vi "SetSubMenuIconType.vi"(8 "error in (no error)":errorcluster, 10 "SubMenuIcon":T1, 11 "Menu in":refnum<class "Menu.lvclass">) -> (0 "error out":errorcluster, 3 "Menu out":refnum<class "Menu.lvclass">)   [LabVIEW 2021, in "Menu.lvlib" / "Menu.lvclass"]
uses:
  Menu.lvclass
  SubMenuIcon.ctl
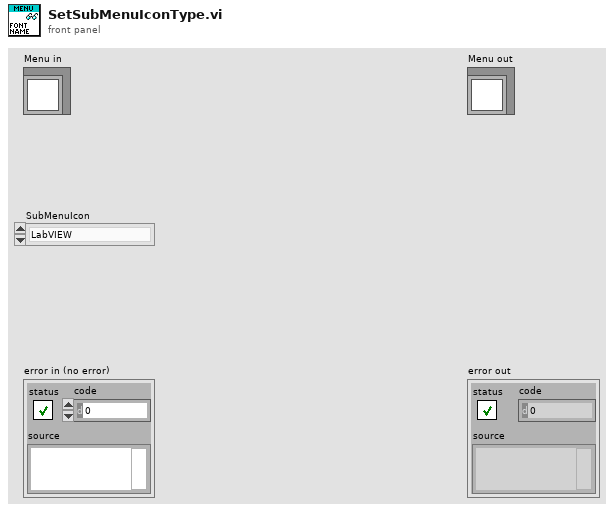
[diagram p1: front panel]
types:
  T1 = typedef "Menu.lvlib/Menu.lvclass/SubMenuIcon.ctl" = enum16{"LabVIEW", "Windows", "Custom"}
  T2 = typedef "Menu.lvlib/Menu.lvclass/Data.ctl" = cluster{"MenuMap":map{string, T3}, "PictRef":refnum<vi>, "MenuSelectionEvent":refnum<user-event>, "TopMenuSpacing":i32, "MenuSpacing":i32, "CloseEvent":refnum<user-event>, "TR_ManageMenuRef":refnum<vi>, "MenuColors":T5, "RTMPath":path, "RTMVIReference":refnum<vi>, "RTMMenuReference":refnum<k9>, "CtlRef":refnum<vi>, "User-Specified Font":refnum<class "Font.lvclass">, "Desired Font":enum16{"User-specified Font", "Application Font", "System Font", "Dialog Font"}, "SubMenuIcon":T1, "SubMenuIconClosed":refnum<class "Picture2D.lvclass">, "SubMenuIconOpened":refnum<class "Picture2D.lvclass">}
  T3 = typedef "Menu.lvlib/Menu.lvclass/MenuItems.ctl" = cluster{"Item Name":string, "Short Cut":T4, "Checked":bool, "Enable":bool, "After item":string, "Item Tags":string[], "Item Names":string[], "Picture":refnum<class "Image.lvclass">, "Hilite Picture":refnum<class "Image.lvclass">, "Displayed":bool}
  T4 = typedef "LVMenuShortCut.ctl" = cluster{"Include Shift Key?":bool, "Include Ctrl Key?":bool, "Shortcut Key":string}
  T5 = typedef "Menu.lvlib/Menu.lvclass/MenuColors.ctl" = cluster{"Text":refnum<class "Color.lvclass">, "HiliteText":refnum<class "Color.lvclass">, "Background":refnum<class "Color.lvclass">, "BorderColor":refnum<class "Color.lvclass">, "Hilite":refnum<class "Color.lvclass">}
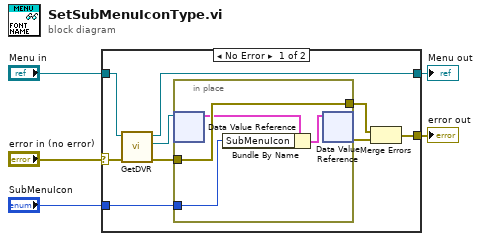
[diagram p0: block diagram]
diagram:
  n1 = case shown="No Error" "error in (no error)" {
    selector: "error in (no error)" -> [w14 w20]
    tunnel: [w8 w20] -> w4
    tunnel: [w12 w19] -> w2
    tunnel: "Menu in" -> [w13 w19]
    tunnel: "SubMenuIcon" -> [w6 _]
    frame No Error {
      n2 = call "GetDVR.vi"("error in (no error)"=w14, "Menu in"=w13) -> ("error out"=w9:errorcluster, "DVR"=w7:refnum<data-value>, "Menu out"=w12:refnum<class "Menu.lvclass">)  [unwired: 7 in]
      n3 = in-place {
        in-place-border: w9 -> [w18]
        in-place-border: [w18] -> w10
        in-place-border: w6 -> [w15]
        n4 = in-place-dvr #1(w7) -> (w17:T2)  [unwired: 1 out]
        n5 = Bundle By Name(cluster=w17, "SubMenuIcon"=w15) -> (w16:T2)
        n6 = in-place-dvr #1(w16) -> (w11:errorcluster)  [unwired: 1 out]
      }
      n7 = Merge Errors(w10, w11) -> (w8:errorcluster)
    }
    frame Error {
    }
  }
  "error out" <- w4
  "Menu out" <- w2
